vi "Messdaten sammeln.vi"(8 "error in (no error)":errorcluster caption="Fehler (Eingang, kein Fehler)", 11 "Gasindex":i32[](array[numeric])) -> (0 "error out":errorcluster caption="Fehler (Ausgang)", 3 "Messdaten":sgl[](array[numeric]))   [LabVIEW 2020, in "EPA 1065.lvlib" / "Chiller NO2 1065-376.lvlib"]
uses:
  Chiller NO2 1065-376.lvlib
  Messdaten/Aktionen FGV Messdaten.ctl
  Seiten/FT-IR/Aktionen EVID-Codes.ctl
  Seiten/FT-IR/FGV FT-IR Aktionen.ctl
  Messdaten/Gewichtung (Stichprobe).ctl
  Messdaten/Messdaten.lvlib
  Seiten/FT-IR/FT-IR.lvlib
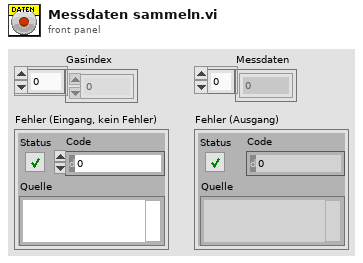
[diagram p1: front panel]
types:
  T1 = typedef "Messdaten.lvlib/Gewichtung (Stichprobe).ctl" = enum16{"Sample", "Population"}
  T2 = typedef "FT-IR.lvlib/FGV FT-IR Aktionen.ctl" = enum16{"lesen", "NOG setzen", "NOS setzen", "Initialisieren", "speichern", "ALLES setzen", "FT-IR Spektrum loggen", "Komm Stoppen", "Spektrum LogKonfig"}
  T3 = typedef "FT-IR.lvlib/Aktionen EVID-Codes.ctl" = enum16{"lesen", "setzen", "laden", "speichern", "1Hz/5Hz", "Smoothing", "Rolling Average"}
  T4 = typedef "Messdaten.lvlib/Aktionen FGV Messdaten.ctl" = enum16{"lesen", "schreiben", "löschen", "Mittelwerte", "Komponente"}
  T5 = typedef "FT-IR.lvlib/1Hz-5Hz Geraet.ctl" = u16
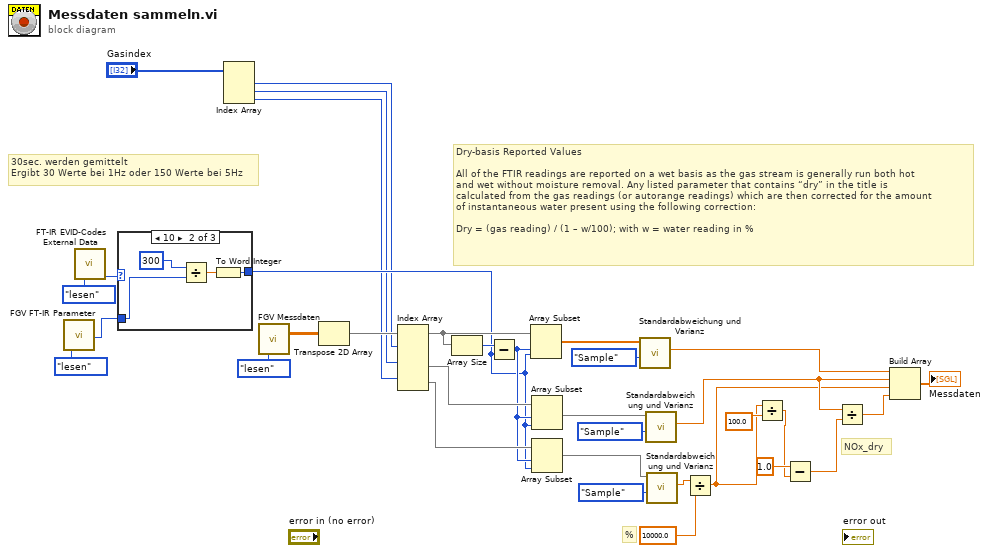
[diagram p0: block diagram]
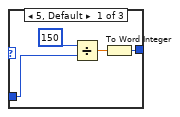
[diagram p2: hidden frame]
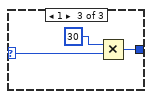
[diagram p3: hidden frame]
diagram:
  # "%"
  # "NOx_dry"
  # "Dry-basis Reported Values\n\nAll of the FTIR readings are reported on a wet basis as the gas stream is generally run both hot\nand wet without moisture removal. Any listed parameter that contains “dry” in the title is\ncalculated from the gas readings (or autorange readings) which are then corrected for the amount\nof instantaneous water present using the following correction:\n\nDry = (gas reading) / (1 – w/100); with w = water reading in %"
  # "30sec. werden gemittelt\nErgibt 30 Werte bei 1Hz oder 150 Werte bei 5Hz"
  n1 = call "FGV FT-IR Parameter.vi"("Aktion"=FGV_FT-IR_Aktionen."lesen") -> ("NoOfScan"=w29:u32)  [unwired: 11 in, 7 out]
  n2 = call "FT-IR EVID-Codes External Data.vi"("Aktionen"=Aktionen_EVID-Codes."lesen") -> ("1Hz/5Hz Gerät"=w30:T5)  [unwired: 9 in, 5 out]
  n3 = case shown="10" w30 {
    selector: w30 -> [_ _ w43]
    tunnel: [w35 w39 w44] -> w20
    tunnel: w29 -> [w37 w41 _]
    frame 5, Default {
      n4 = Divide(x=150, y=w37) -> (x/y=w36:dbl)
      n5 = To Word Integer(number=w36) -> (16bit integer=w35:i16)
    }
    frame 10 {
      n6 = Divide(x=300, y=w41) -> (x/y=w40:dbl)
      n7 = To Word Integer(number=w40) -> (16bit integer=w39:i16)
    }
    frame 1 {
      n8 = Multiply(x=30, y=w43) -> (x*y=w44:i32)
    }
  }
  n9 = Index Array(array="Gasindex") -> (element #1=w12:i32, element #2=w11:i32, element #3=w10:i32)  [unwired: 3 in]
  n10 = call "FGV Messdaten.vi"("Aktionen"=Aktionen_FGV_Messdaten."lesen") -> ("Messdaten"=w33:sgl[][])  [unwired: 6 in, 8 out]
  n11 = Transpose 2D Array(2D array=w33) -> (transposed array=w28:sgl[][])
  n12 = Index Array(array=w28, index (row) #1=w12, index (row) #2=w11, index (row) #3=w10) -> (element #1=w24:sgl[], element #2=w23:sgl[], element #3=w22:sgl[])  [unwired: 3 in]
  n13 = Array Size(array=w24) -> (size(s)=w27:i32)
  n14 = Subtract(x=w27, y=w20) -> (x-y=w21:i32)
  n15 = Array Subset(array=w24, index=w21, length=w20) -> (w25:sgl[])
  n16 = Array Subset(array=w23, index=w21, length=w20) -> (w16:sgl[])
  n17 = Array Subset(array=w22, index=w21, length=w20) -> (w17:sgl[])
  n18 = call "Standardabweichung und Varianz.vi"("Gewichtung (Stichprobe)"=Gewichtung_(Stichprobe)."Sample", "X"=w25) -> ("Mittelwert"=w15:sgl)  [unwired: 7 in, 2 out]
  n19 = call "Standardabweichung und Varianz.vi"("Gewichtung (Stichprobe)"=Gewichtung_(Stichprobe)."Sample", "X"=w16) -> ("Mittelwert"=w6:sgl)  [unwired: 7 in, 2 out]
  n20 = call "Standardabweichung und Varianz.vi"("Gewichtung (Stichprobe)"=Gewichtung_(Stichprobe)."Sample", "X"=w17) -> ("Mittelwert"=w3:sgl)  [unwired: 7 in, 2 out]
  n21 = Divide(x=w3, y=sgl 10000.0) -> (x/y=w2:sgl)
  n22 = Divide(x=w2, y=sgl 100.0) -> (x/y=w7:sgl)
  n23 = Subtract(x=1.0, y=w7) -> (x-y=w5:dbl)
  n24 = Divide(x=w6, y=w5) -> (x/y=w4:dbl)
  n25 = Build Array(w15, w6, w2, w4) -> (→"Messdaten":dbl[])
